vi "CleanUp.vi"(8 "error in (no error)":errorcluster, 11 "object in":refnum<class "JuPyter_Client.lvclass">) -> (0 "error out":errorcluster, 3 "object out":refnum<class "JuPyter_Client.lvclass">)   [LabVIEW 2018, in "JuPyter_Client.lvclass"]
uses:
  JuPyter_Client.lvclass
  JuPyter_Client.lvclass/JuPyter_Client.ctl
  <vilib>/addons/zeromq/zmq_context.lvclass
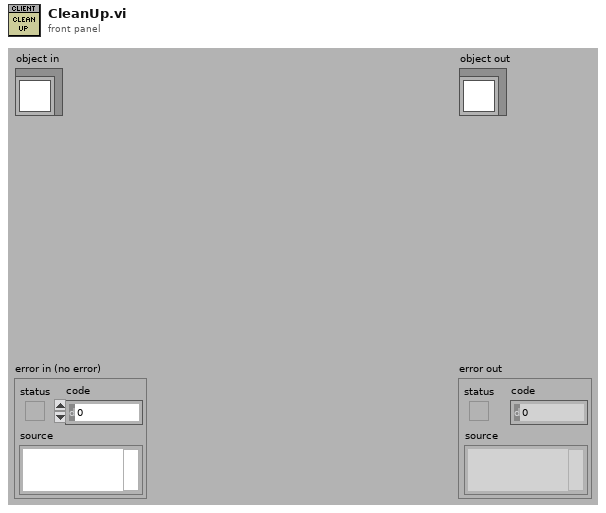
[diagram p1: front panel]
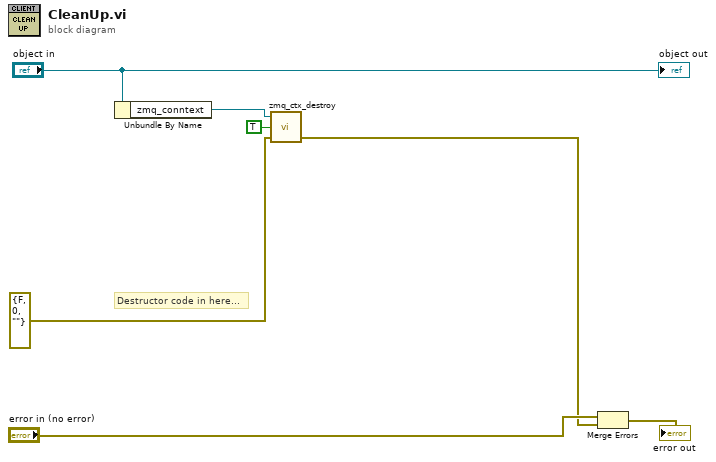
[diagram p0: block diagram]
diagram:
  # "Destructor code in here..."
  n1 = Unbundle By Name("object in") -> ("zmq_conntext"=w4:refnum<class "zmq_context.lvclass">)
  n2 = call <vilib>:"zmq_ctx_destroy.vi"("error in"=errorcluster {"status"=FALSE, "code"=0, "source"=""} ("error in (no error)"), "reap? (F)"=TRUE, "context in"=w4) -> ("error out"=w2:errorcluster)  [unwired: 2 in]
  n3 = Merge Errors("error in (no error)", w2) -> (→"error out":errorcluster)
  "object out" <- "object in"
